vi "LAC Cmd102_Individual Setting.vi"(6 "R/W (F:Read)":bool, 7 "timeout(ms)":u32=500, 8 "error in":errorcluster, 9 "set_val":dbl, 10 "item_code":T1=enum."Center of gravity calculation method", 11 "VISA name in":refnum<visa-resource-name>) -> (0 "error out":errorcluster, 1 "read buffer":string, 3 "VISA name out":refnum<visa-resource-name>)   [LabVIEW 2014]
uses:
  TypeDef/H410 ItemCode TypeDef.ctl
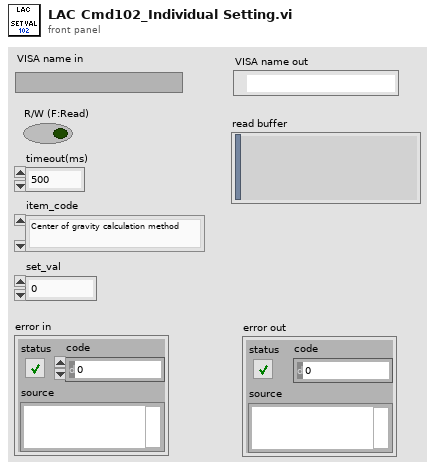
[diagram p1: front panel]
types:
  T1 = typedef "H410 ItemCode TypeDef.ctl" = enum16{"Luminance Binary level", "Luminance Noise level", "Luminance upper limit", "Luminance lower limit", "Luminance judgment mode", "Judgment type", "Circle-radius", "Rectangular-XL", "Rectangular-XH", "Rectangular-YH", "Rectangular-YL", "Circle2-radius", "Offset-X", "Offset-Y", "Label meas. mode", "Numbering", "Judgment label", "Max No. of spot", "Center of gravity calculation method", "Average", "Effective spot size mode", "Effective spot pixel upper limit", "Effective spot pixel lower limit"}
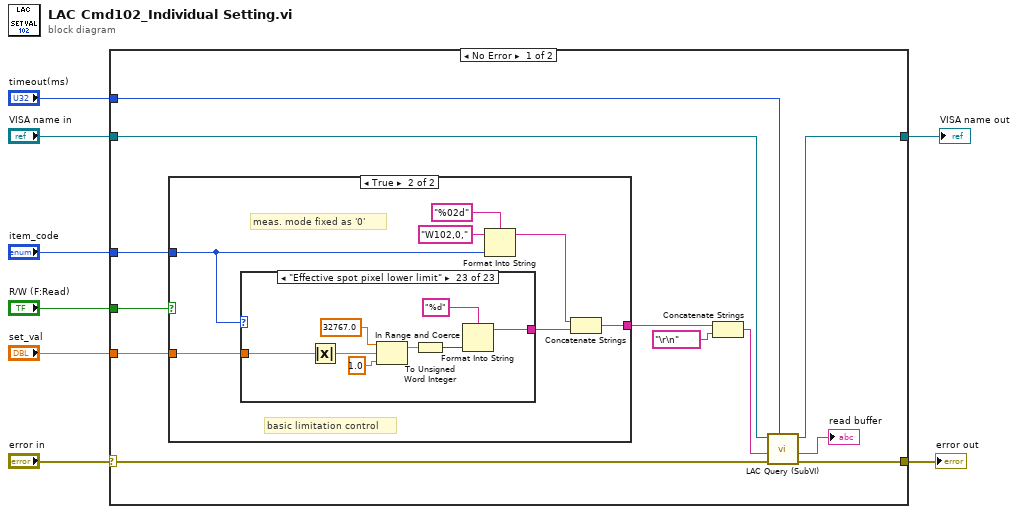
[diagram p0: block diagram]
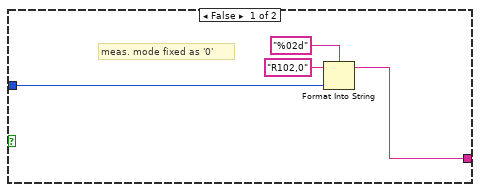
[diagram p2: hidden frame]
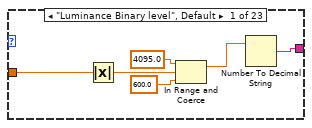
[diagram p3: hidden frame]
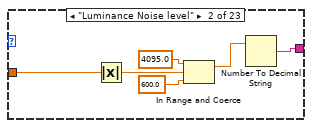
[diagram p4: hidden frame]
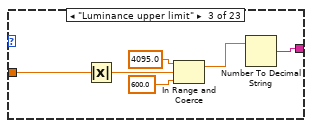
[diagram p5: hidden frame]
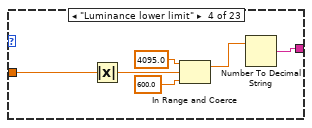
[diagram p6: hidden frame]
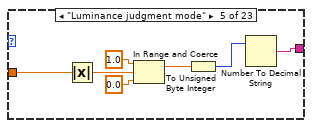
[diagram p7: hidden frame]
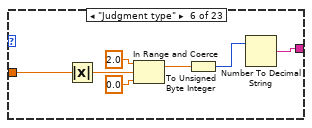
[diagram p8: hidden frame]
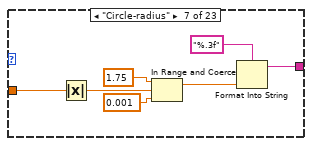
[diagram p9: hidden frame]
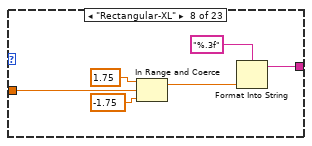
[diagram p10: hidden frame]
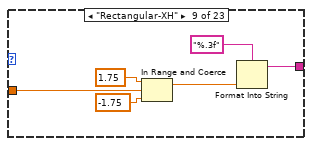
[diagram p11: hidden frame]
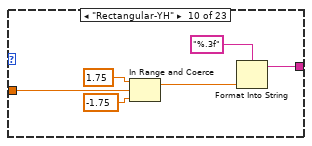
[diagram p12: hidden frame]
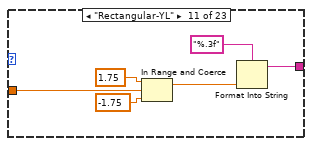
[diagram p13: hidden frame]
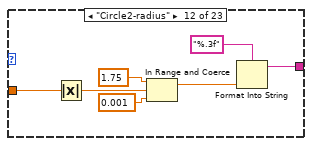
[diagram p14: hidden frame]
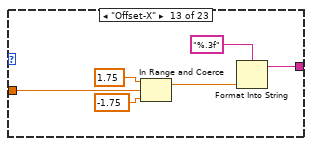
[diagram p15: hidden frame]
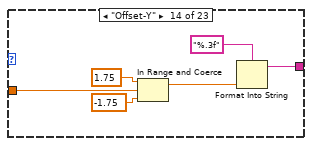
[diagram p16: hidden frame]
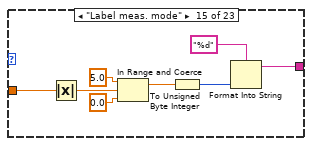
[diagram p17: hidden frame]
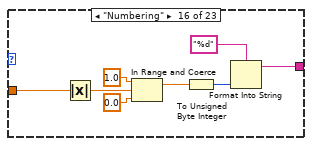
[diagram p18: hidden frame]
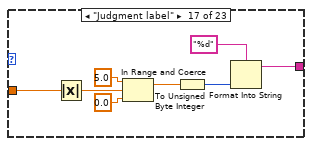
[diagram p19: hidden frame]
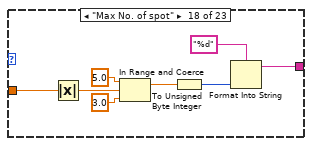
[diagram p20: hidden frame]
diagram:
  n1 = case shown="No Error" "error in" {
    selector: "error in" -> [w15 w193]
    tunnel: "VISA name in" -> [w17 w192]
    tunnel: [w20 w192] -> w7
    tunnel: [w18 w193] -> w6
    tunnel: "timeout(ms)" -> [w16 _]
    tunnel: "item_code" -> [w9 _]
    tunnel: "R/W (F:Read)" -> [w12 _]
    tunnel: "set_val" -> [w10 _]
    frame No Error {
      n2 = case shown="True" w12 {
        tunnel: [w21 w29] -> w11
        tunnel: w10 -> [_ w31]
        tunnel: w9 -> [w22 w26]
        frame False {
          # "meas. mode fixed as '0'"
          n3 = Format Into String(format string="%02d", initial string="R102,0" ("string"), w22) -> (resulting string=w21:string)  [unwired: 1 in, 1 out]
        }
        frame True {
          # "basic limitation control"
          # "meas. mode fixed as '0'"
          n4 = case shown="\"Effective spot pixel lower limit\"" w26 {
            tunnel: w31 -> [w37 w39 w45 w51 w57 w65 w73 w78 w83 w90 w96 w101 w109 w115 w123 w133 w137 w145 w153 w161 w169 w177 w184]
            tunnel: [w36 w38 w44 w50 w58 w64 w72 w77 w84 w89 w95 w103 w108 w114 w122 w128 w136 w144 w152 w160 w168 w176 w185] -> w30
            frame "Luminance Binary level", Default {
              n5 = Absolute Value(x=w37) -> (abs(x)=w32:dbl)
              n6 = In Range and Coerce(upper limit=4095.0 ("y"), x=w32, lower limit=600.0) -> (coerced(x)=w33:dbl)  [unwired: 1 out]
              n7 = Number To Decimal String(number=w33) -> (decimal integer string=w36:string)  [unwired: 1 in]
            }
            frame "Luminance Noise level" {
              n8 = Absolute Value(x=w39) -> (abs(x)=w40:dbl)
              n9 = In Range and Coerce(upper limit=4095.0 ("y"), x=w40, lower limit=600.0) -> (coerced(x)=w41:dbl)  [unwired: 1 out]
              n10 = Number To Decimal String(number=w41) -> (decimal integer string=w38:string)  [unwired: 1 in]
            }
            frame "Luminance upper limit" {
              n11 = Absolute Value(x=w45) -> (abs(x)=w46:dbl)
              n12 = In Range and Coerce(upper limit=4095.0 ("y"), x=w46, lower limit=600.0) -> (coerced(x)=w47:dbl)  [unwired: 1 out]
              n13 = Number To Decimal String(number=w47) -> (decimal integer string=w44:string)  [unwired: 1 in]
            }
            frame "Luminance lower limit" {
              n14 = Absolute Value(x=w51) -> (abs(x)=w52:dbl)
              n15 = In Range and Coerce(upper limit=4095.0 ("y"), x=w52, lower limit=600.0) -> (coerced(x)=w53:dbl)  [unwired: 1 out]
              n16 = Number To Decimal String(number=w53) -> (decimal integer string=w50:string)  [unwired: 1 in]
            }
            frame "Luminance judgment mode" {
              n17 = Absolute Value(x=w57) -> (abs(x)=w59:dbl)
              n18 = In Range and Coerce(upper limit=1.0 ("y"), x=w59, lower limit=0.0) -> (coerced(x)=w60:dbl)  [unwired: 1 out]
              n19 = To Unsigned Byte Integer(number=w60) -> (unsigned 8bit integer=w56:u8)
              n20 = Number To Decimal String(number=w56) -> (decimal integer string=w58:string)  [unwired: 1 in]
            }
            frame "Judgment type" {
              n21 = Absolute Value(x=w65) -> (abs(x)=w66:dbl)
              n22 = In Range and Coerce(upper limit=2.0 ("y"), x=w66, lower limit=0.0) -> (coerced(x)=w67:dbl)  [unwired: 1 out]
              n23 = To Unsigned Byte Integer(number=w67) -> (unsigned 8bit integer=w63:u8)
              n24 = Number To Decimal String(number=w63) -> (decimal integer string=w64:string)  [unwired: 1 in]
            }
            frame "Circle-radius" {
              n25 = Absolute Value(x=w73) -> (abs(x)=w74:dbl)
              n26 = In Range and Coerce(upper limit=1.75 ("y"), x=w74, lower limit=0.001) -> (coerced(x)=w71:dbl)  [unwired: 1 out]
              n27 = Format Into String(format string="%.3f", w71) -> (resulting string=w72:string)  [unwired: 2 in, 1 out]
            }
            frame "Rectangular-XL" {
              n28 = In Range and Coerce(upper limit=1.75 ("y"), x=w78, lower limit=-1.75) -> (coerced(x)=w80:dbl)  [unwired: 1 out]
              n29 = Format Into String(format string="%.3f", w80) -> (resulting string=w77:string)  [unwired: 2 in, 1 out]
            }
            frame "Rectangular-XH" {
              n30 = In Range and Coerce(upper limit=1.75 ("y"), x=w83, lower limit=-1.75) -> (coerced(x)=w86:dbl)  [unwired: 1 out]
              n31 = Format Into String(format string="%.3f", w86) -> (resulting string=w84:string)  [unwired: 2 in, 1 out]
            }
            frame "Rectangular-YH" {
              n32 = In Range and Coerce(upper limit=1.75 ("y"), x=w90, lower limit=-1.75) -> (coerced(x)=w92:dbl)  [unwired: 1 out]
              n33 = Format Into String(format string="%.3f", w92) -> (resulting string=w89:string)  [unwired: 2 in, 1 out]
            }
            frame "Rectangular-YL" {
              n34 = In Range and Coerce(upper limit=1.75 ("y"), x=w96, lower limit=-1.75) -> (coerced(x)=w98:dbl)  [unwired: 1 out]
              n35 = Format Into String(format string="%.3f", w98) -> (resulting string=w95:string)  [unwired: 2 in, 1 out]
            }
            frame "Circle2-radius" {
              n36 = Absolute Value(x=w101) -> (abs(x)=w102:dbl)
              n37 = In Range and Coerce(upper limit=1.75 ("y"), x=w102, lower limit=0.001) -> (coerced(x)=w105:dbl)  [unwired: 1 out]
              n38 = Format Into String(format string="%.3f", w105) -> (resulting string=w103:string)  [unwired: 2 in, 1 out]
            }
            frame "Offset-X" {
              n39 = In Range and Coerce(upper limit=1.75 ("y"), x=w109, lower limit=-1.75) -> (coerced(x)=w111:dbl)  [unwired: 1 out]
              n40 = Format Into String(format string="%.3f", w111) -> (resulting string=w108:string)  [unwired: 2 in, 1 out]
            }
            frame "Offset-Y" {
              n41 = In Range and Coerce(upper limit=1.75 ("y"), x=w115, lower limit=-1.75) -> (coerced(x)=w117:dbl)  [unwired: 1 out]
              n42 = Format Into String(format string="%.3f", w117) -> (resulting string=w114:string)  [unwired: 2 in, 1 out]
            }
            frame "Label meas. mode" {
              n43 = Absolute Value(x=w123) -> (abs(x)=w120:dbl)
              n44 = In Range and Coerce(upper limit=5.0 ("y"), x=w120, lower limit=0.0) -> (coerced(x)=w125:dbl)  [unwired: 1 out]
              n45 = To Unsigned Byte Integer(number=w125) -> (unsigned 8bit integer=w121:u8)
              n46 = Format Into String(format string="%d", w121) -> (resulting string=w122:string)  [unwired: 2 in, 1 out]
            }
            frame "Numbering" {
              n47 = Absolute Value(x=w133) -> (abs(x)=w132:dbl)
              n48 = In Range and Coerce(upper limit=1.0 ("y"), x=w132, lower limit=0.0) -> (coerced(x)=w129:dbl)  [unwired: 1 out]
              n49 = To Unsigned Byte Integer(number=w129) -> (unsigned 8bit integer=w131:u8)
              n50 = Format Into String(format string="%d", w131) -> (resulting string=w128:string)  [unwired: 2 in, 1 out]
            }
            frame "Judgment label" {
              n51 = Absolute Value(x=w137) -> (abs(x)=w141:dbl)
              n52 = In Range and Coerce(upper limit=5.0 ("y"), x=w141, lower limit=0.0) -> (coerced(x)=w138:dbl)  [unwired: 1 out]
              n53 = To Unsigned Byte Integer(number=w138) -> (unsigned 8bit integer=w140:u8)
              n54 = Format Into String(format string="%d", w140) -> (resulting string=w136:string)  [unwired: 2 in, 1 out]
            }
            frame "Max No. of spot" {
              n55 = Absolute Value(x=w145) -> (abs(x)=w149:dbl)
              n56 = In Range and Coerce(upper limit=5.0 ("y"), x=w149, lower limit=3.0) -> (coerced(x)=w146:dbl)  [unwired: 1 out]
              n57 = To Unsigned Byte Integer(number=w146) -> (unsigned 8bit integer=w148:u8)
              n58 = Format Into String(format string="%d", w148) -> (resulting string=w144:string)  [unwired: 2 in, 1 out]
            }
            frame "Center of gravity calculation method" {
              n59 = Absolute Value(x=w153) -> (abs(x)=w157:dbl)
              n60 = In Range and Coerce(upper limit=2.0 ("y"), x=w157, lower limit=0.0) -> (coerced(x)=w154:dbl)  [unwired: 1 out]
              n61 = To Unsigned Byte Integer(number=w154) -> (unsigned 8bit integer=w156:u8)
              n62 = Format Into String(format string="%d", w156) -> (resulting string=w152:string)  [unwired: 2 in, 1 out]
            }
            frame "Average" {
              n63 = Absolute Value(x=w161) -> (abs(x)=w165:dbl)
              n64 = In Range and Coerce(upper limit=4.0 ("y"), x=w165, lower limit=0.0) -> (coerced(x)=w162:dbl)  [unwired: 1 out]
              n65 = To Unsigned Byte Integer(number=w162) -> (unsigned 8bit integer=w164:u8)
              n66 = Format Into String(format string="%d", w164) -> (resulting string=w160:string)  [unwired: 2 in, 1 out]
            }
            frame "Effective spot size mode" {
              n67 = Absolute Value(x=w169) -> (abs(x)=w173:dbl)
              n68 = In Range and Coerce(upper limit=1.0 ("y"), x=w173, lower limit=0.0) -> (coerced(x)=w170:dbl)  [unwired: 1 out]
              n69 = To Unsigned Byte Integer(number=w170) -> (unsigned 8bit integer=w172:u8)
              n70 = Format Into String(format string="%d", w172) -> (resulting string=w168:string)  [unwired: 2 in, 1 out]
            }
            frame "Effective spot pixel upper limit" {
              n71 = Absolute Value(x=w177) -> (abs(x)=w181:dbl)
              n72 = In Range and Coerce(upper limit=32767.0 ("y"), x=w181, lower limit=1.0) -> (coerced(x)=w178:dbl)  [unwired: 1 out]
              n73 = To Unsigned Word Integer(number=w178) -> (unsigned 16bit integer=w180:u16)
              n74 = Format Into String(format string="%d", w180) -> (resulting string=w176:string)  [unwired: 2 in, 1 out]
            }
            frame "Effective spot pixel lower limit" {
              n75 = Absolute Value(x=w184) -> (abs(x)=w189:dbl)
              n76 = In Range and Coerce(upper limit=32767.0 ("y"), x=w189, lower limit=1.0) -> (coerced(x)=w186:dbl)  [unwired: 1 out]
              n77 = To Unsigned Word Integer(number=w186) -> (unsigned 16bit integer=w188:u16)
              n78 = Format Into String(format string="%d", w188) -> (resulting string=w185:string)  [unwired: 2 in, 1 out]
            }
          }
          n79 = Format Into String(format string="%02d", initial string="W102,0," ("string"), w26) -> (resulting string=w25:string)  [unwired: 1 in, 1 out]
          n80 = Concatenate Strings(w25, w30) -> (w29:string)
        }
      }
      n81 = Concatenate Strings(w11, "\r\n" ("write buffer")) -> (w13:string)
      n82 = call "LAC Query (SubVI).vi"("timeout(ms)"=w16, "error in"=w15, "Command"=w13, "VISA name in"=w17) -> ("error out"=w18:errorcluster, "read buffer"=→"read buffer":string, "VISA name out"=w20:refnum<visa-resource-name>)  [unwired: 5 in]
    }
    frame Error {
    }
  }
  "VISA name out" <- w7
  "error out" <- w6
